vi "GetLimsTestsForBench.vi"(8 "error in (no error)":errorcluster, 9 "creation date":timestamp, 10 "workbench":string, 11 "ByteQXAPIBase in":refnum<class "ByteQXAPIBase.lvclass">) -> (0 "error out":errorcluster, 2 "list of tests":T1[](array[typedef]), 3 "ByteQXAPIBase out":refnum<class "ByteQXAPIBase.lvclass">)   [LabVIEW 2019, in "ByteQXWebAPI.lvlib" / "ByteQXAPIBase.lvclass"]
doc: "Request the list of Tests based on Workstation and Creation date (optional)"
uses:
  ByteQXAPIBase.lvclass
  TypeDef/Test.ctl
  TypeDef/Asset.ctl
  Private/module.ctl
  ByteQXAPIBase.lvclass/ByteQXAPIBase.ctl
  <vilib>/Bytelabs/ByteREST/ByteRESTClass/ByteRESTBase/RESTBase.lvclass
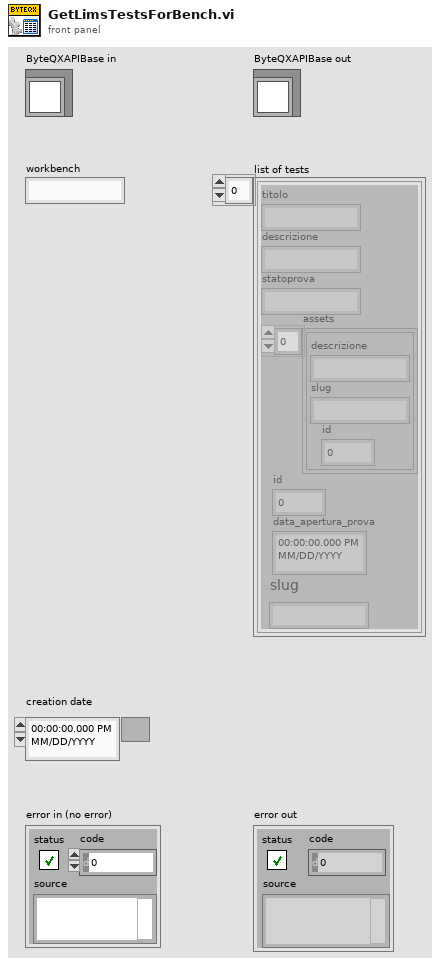
[diagram p1: front panel]
types:
  T1 = typedef "ByteQXWebAPI.lvlib/ByteQXAPIBase.lvclass/Test.ctl" = cluster{"titolo":string, "descrizione":string, "statoprova":string, "assets":T2[], "id":i32, "data_apertura_prova":timestamp, "slug":string}
  T2 = typedef "ByteQXWebAPI.lvlib/ByteQXAPIBase.lvclass/Asset.ctl" = cluster{"descrizione":string, "slug":string, "id":i32}
  T3 = typedef "ByteQXWebAPI.lvlib/ByteQXAPIBase.lvclass/module.ctl" = enum16{"gs", "tms", "data"}
  T4 = cluster{"titolo":string, "descrizione":string, "statoprova":string, "assets":cluster{"descrizione":string, "slug":string, "id":i32}[], "data_apertura_prova":string, "id":i32, "slug":string}[]
  T5 = cluster{"descrizione":string, "slug":string, "id":i32}[]
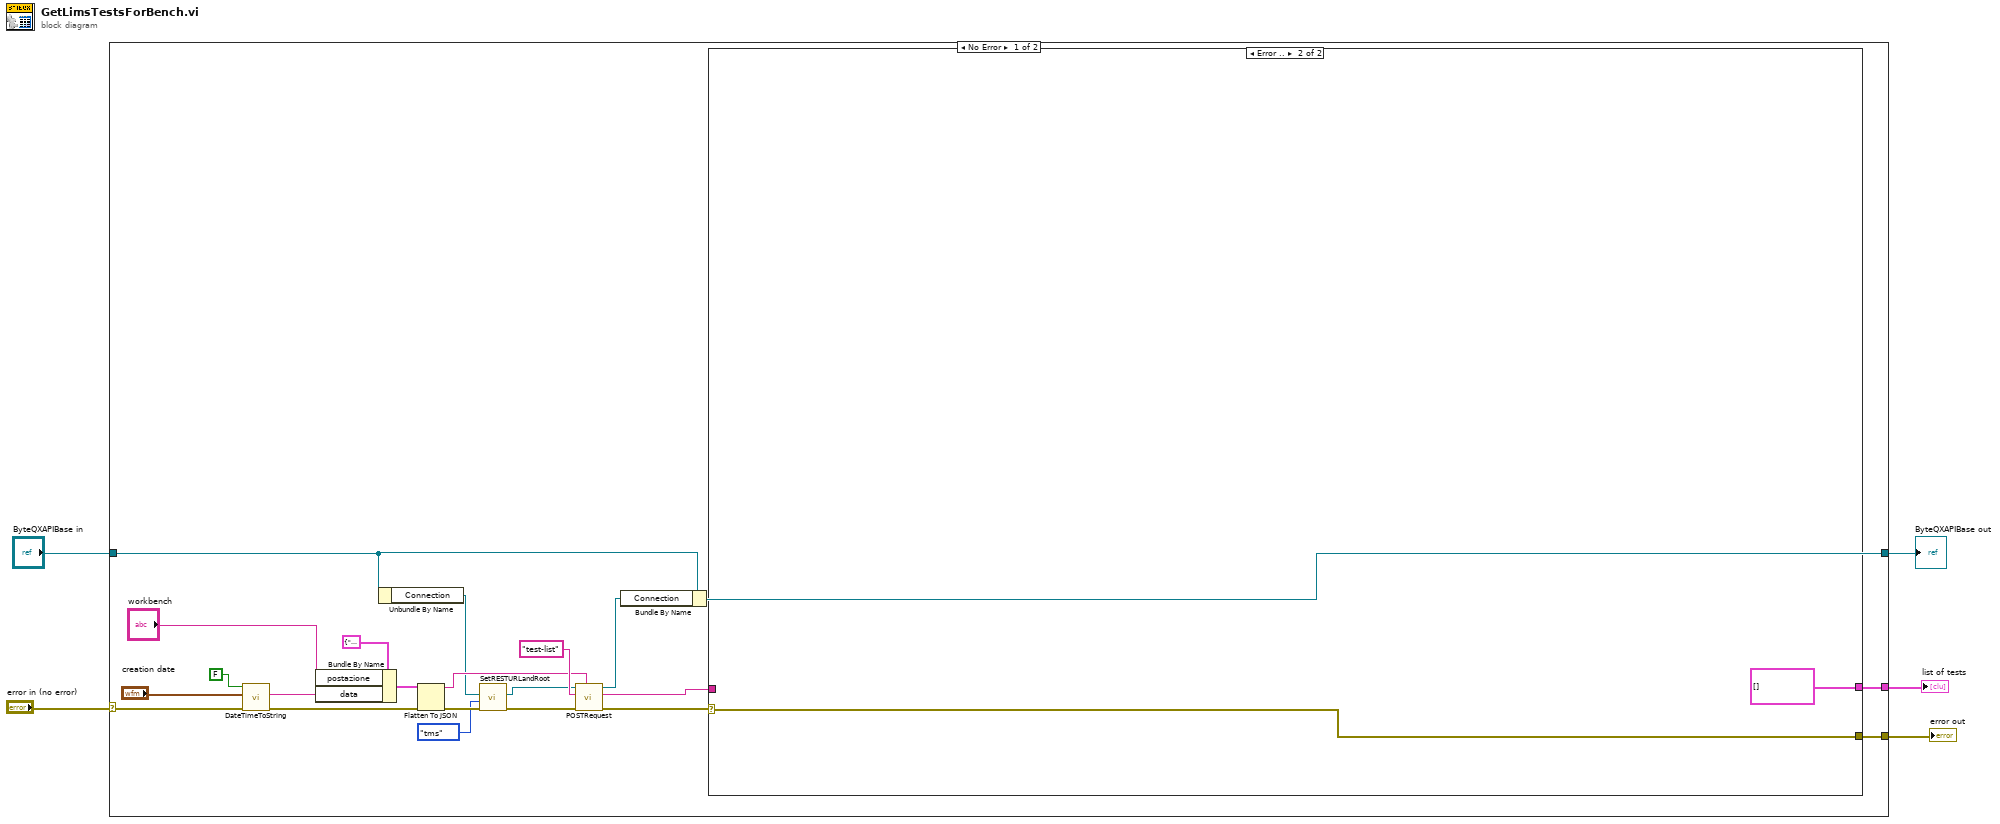
[diagram p0: block diagram]
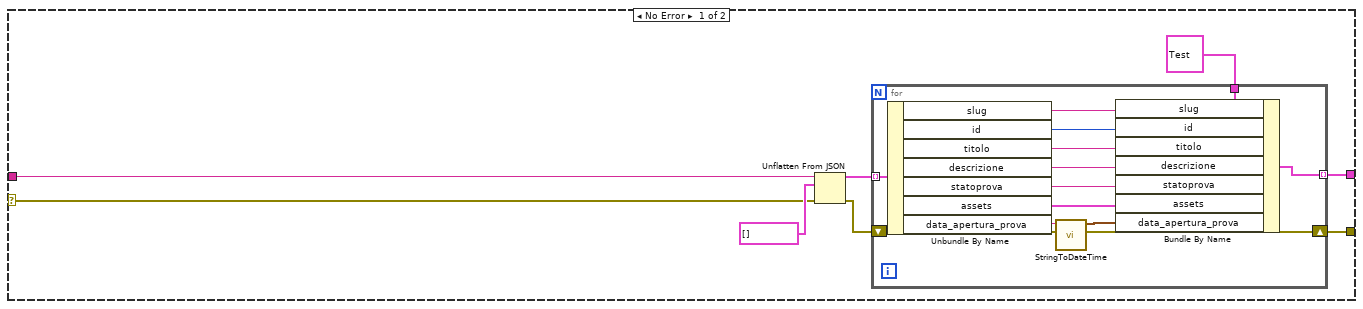
[diagram p2: hidden frame]
diagram:
  n1 = case shown="No Error" "error in (no error)" {
    selector: "error in (no error)" -> [w16 w52]
    tunnel: [w22 w52] -> w4
    tunnel: [w26 w51] -> w2
    tunnel: "ByteQXAPIBase in" -> [w20 w51]
    tunnel: [w21 _] -> w1
    frame No Error {
      n2 = call "DateTimeToString.vi"("error in"=w16, "current time"="creation date", "include Time?"=FALSE ("Time")) -> ("error out"=w17:errorcluster, "date string"=w15:string)  [unwired: 7 in]
      n3 = Bundle By Name(cluster=cluster{"postazione":string, "data":string} {"postazione"="", "data"=""} ("Request"), "postazione"="workbench", "data"=w15) -> (w18:cluster{"postazione":string, "data":string})
      n4 = Unbundle By Name(w20) -> ("Connection"=w8:refnum<class "RESTBase.lvclass">)
      n5 = Flatten To JSON(anything=w18, error in (no error)=w17) -> (JSON string=w24:string, 11:w10:errorcluster)  [unwired: 1 in]
      n6 = call "SetRESTURLandRoot.vi"("error in (no error)"=w10, "module"=module."tms", "ByteREST in"=w8) -> ("error out"=w9:errorcluster, "ByteREST out"=w7:refnum<class "RESTBase.lvclass">)  [unwired: 7 in]
      n7 = call-dynamic "POSTRequest.vi"("Body in"=w24, "error in (no error)"=w9, "Request"="test-list", "ByteRESTBase in"=w7) -> ("error out"=w12:errorcluster, "Body"=w23:string, "ByteRESTBase out"=w27:refnum<class "RESTBase.lvclass">)  [unwired: 4 in, 1 out]
      n8 = Bundle By Name(cluster=w20, "Connection"=w27) -> (w26:refnum<class "ByteQXAPIBase.lvclass">)
      n9 = case shown="Error .." w12 {
        selector: w12 -> [w28 w50]
        tunnel: w23 -> [w35 _]
        tunnel: [w31 w50] -> w22
        tunnel: [w30 T1[] []] -> w21
        frame No Error {
          n10 = Unflatten From JSON(JSON string=w35, type and defaults=T4 [], error in (no error)=w28) -> (value=w33:T4, error out=w32:errorcluster)  [unwired: 4 in]
          n11 = for {
            tunnel: w33 -> [w48] mode=indexing
            tunnel: T1 {"titolo"="", "descrizione"="", "statoprova"="", "assets"=[], "id"=0, "data_apertura_prova"=timestamp(0 s since 1904-01-01), "slug"=""} ("ByteQXWebAPI.lvlib:ByteQXAPIBase.lvclass:Test") -> [w47]
            shift-right: [w37] -> w31
            shift-left: w32 -> [w38]
            tunnel: [w41] -> w30 mode=indexing
            n12 = Unbundle By Name(w48) -> ("slug"=w36:string, "id"=w46:i32, "titolo"=w45:string, "descrizione"=w44:string, "statoprova"=w43:string, "assets"=w42:T5, "data_apertura_prova"=w40:string)
            n13 = call "StringToDateTime.vi"("error in (no error)"=w38, "datetime string"=w40) -> ("error out"=w37:errorcluster, "timestamp"=w39:timestamp)  [unwired: 8 in]
            n14 = Bundle By Name(cluster=w47, "slug"=w36, "id"=w46, "titolo"=w45, "descrizione"=w44, "statoprova"=w43, "assets"=w42, "data_apertura_prova"=w39) -> (w41:T1)
          }
        }
        frame Error {
        }
      }
    }
    frame Error {
    }
  }
  "error out" <- w4
  "ByteQXAPIBase out" <- w2
  "list of tests" <- w1
